vi "To String.vi"(6 "Encoding [No encoding]":refnum<class "CConfig Encoding.lvclass">, 7 "Persitant only? [T]":bool=TRUE, 8 "error in (no error)":errorcluster, 11 "Carya Config in":refnum<class "Carya Config.lvclass">) -> (0 "error out":errorcluster, 2 "String":string, 3 "Carya Config out":refnum<class "Carya Config.lvclass">)   [LabVIEW 2013, in "Carya Config.lvclass"]
doc: "Copyright 2018, Carya Automatisering, Wiebe Walstra."
uses:
  Carya Config.lvclass
  CConfig Encoding/CConfig Encoding.lvclass
  Carya Config.lvclass/Carya Config.ctl
  CConfig Object/CConfig Object.lvclass
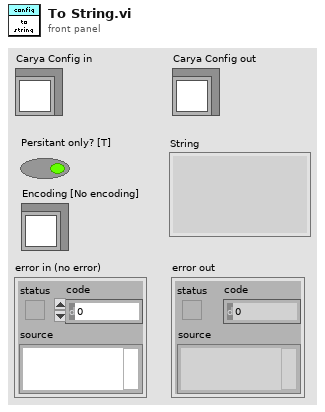
[diagram p1: front panel]
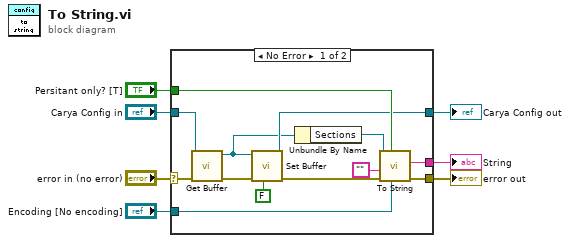
[diagram p0: block diagram]
diagram:
  n1 = case shown="No Error" "error in (no error)" {
    selector: "error in (no error)" -> [w20 w22]
    tunnel: [w9 w22] -> w6
    tunnel: [w18 w21] -> w4
    tunnel: "Carya Config in" -> [w17 w21]
    tunnel: [w16 _] -> w3
    tunnel: "Persitant only? [T]" -> [w19 _]
    tunnel: "Encoding [No encoding]" -> [w8 _]
    frame No Error {
      n2 = call-dynamic "Get Buffer.vi"("error in (no error)"=w20, "Carya Config in"=w17) -> ("error out"=w12:errorcluster, "Config"=w10:refnum<class "Carya Config.lvclass">)  [unwired: 8 in]
      n3 = call-dynamic "Set Buffer.vi"("Set? [T]"=FALSE, "error in (no error)"=w12, "Carya Config"=w10) -> ("error out"=w11:errorcluster, "Carya Config out"=w18:refnum<class "Carya Config.lvclass">)  [unwired: 7 in]
      n4 = Unbundle By Name(w10) -> ("Sections"=w14:refnum<class "CConfig Object.lvclass">)
      n5 = call-dynamic "To String.vi"("Encoding [No encoding]"=w8, "Persitant only?"=w19, "error in (no error)"=w11, "Prev. Newline"="", "Section Object in"=w14) -> ("error out"=w9:errorcluster, "String"=w16:string)  [unwired: 3 in, 2 out]
    }
    frame Error {
    }
  }
  "error out" <- w6
  "Carya Config out" <- w4
  "String" <- w3
